vi "MoveArm.vi"(8 "BackwardValue":dbl=-0.10000000000000014 min=-1.0 max=0.0 step=0.1, 9 "ForwardValue":dbl=0.10000000000000014 min=0.0 max=1.0 step=0.1, 10 "Direction":bool, 11 "Move Or Not":bool) -> ()   [LabVIEW 2013]
doc: "moves the motor forwards or backwards depending on the state of the diretion boolean(true = forwards, false = backwards) input, and will move or turn off the motor according to the move or not boolean input."
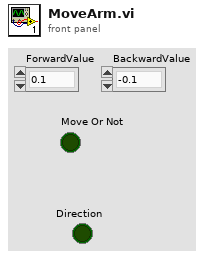
[diagram p1: front panel]
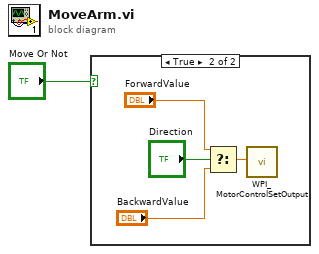
[diagram p0: block diagram]
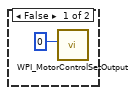
[diagram p2: hidden frame]
diagram:
  n1 = case shown="True" "Move Or Not" {
    frame False {
      n2 = call <vilib>:"WPI_MotorControlSetOutput.vi"("Output"=0) -> ()  [unwired: 8 in, 3 out]
    }
    frame True {
      n3 = Select(t="ForwardValue", s="Direction", f="BackwardValue") -> (s? t:f=w6:dbl)
      n4 = call <vilib>:"WPI_MotorControlSetOutput.vi"("Output"=w6) -> ()  [unwired: 8 in, 3 out]
    }
  }
